vi "Periodic Tasks.vi"(8 "error in":errorcluster) -> ()   [LabVIEW 2018]
doc: "This VI runs in parallel to other tasks. It can contain as many user-defined periodic loops as you need. These can carry out PID or other sorts of timed response."
uses:
  CTL_RangeFinder_Type.ctl
  <vilib>/Rock Robotics/WPI/Utilities/WPI_GetSetVariantRefNum.vi
  Robot Global Data.vi
  <vilib>/Rock Robotics/Network Tables/NT Write Numeric Array.vi
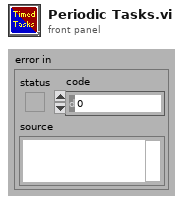
[diagram p1: front panel]
types:
  T1 = typedef "WPI_JoystickDevRef.ctl" = cluster{"Device":T2}
  T2 = typedef "WPI_JoystickDeviceEnum.ctl" = enum16{"USB 0", "USB 1", "USB 2", "USB 3", "USB 4", "USB 5"}
  T3 = typedef "WPI_RobotDriveDevRef.ctl" = cluster{"DevStatus":errorcluster, "Motors[]":T4[], "Square Inputs":bool, "Max Output":dbl}
  T4 = typedef "WPI_MotorControlDeviceRef.ctl" = cluster{"DeviceStatus":errorcluster, "Type":T5, "PWM":cluster{"PWM Channel":T6, "DeadBand":T7}, "CAN":cluster{"Device Number":u8, "SetOutput VI Ref":variant, "GetOutput VI Ref":variant, "Enable VI Ref":variant, "Disable VI Ref":variant, "Data":variant}, "Invert":bool, "DIO PWM":cluster{"PWM \"Enable\" Channel":T6, "DIOChannel":T8, "PWM Rate":dbl}}
  T5 = typedef "WPI_MotorControlType.ctl" = enum16{"PWM", "CAN", "DIO PWM"}
  T6 = typedef "FPGA_DIOPWMChannel.ctl" = enum8{"PWM 0", "PWM 1", "PWM 2", "PWM 3", "PWM 4", "PWM 5", "PWM 6", "PWM 7", "PWM 8", "PWM 9", "PWM MXP 0", "PWM MXP 1", "PWM MXP 2", "PWM MXP 3", "PWM MXP 4", "PWM MXP 5", "PWM MXP 6", "PWM MXP 7", "PWM MXP 8", "PWM MXP 9", "Invalid"}
  T7 = typedef "WPI_PWMDeadband.ctl" = cluster{"Name":string, "maxPositivePwm":i32, "minPositivePwm":i32, "centerPwm":i32, "maxNegativePwm":i32, "minNegativePwm":i32, "angularRange":u16}
  T8 = typedef "FPGA_DIOChannel.ctl" = enum8{"DIO 0", "DIO 1", "DIO 2", "DIO 3", "DIO 4", "DIO 5", "DIO 6", "DIO 7", "DIO 8", "DIO 9", "DIO MXP 0", "DIO MXP 1", "DIO MXP 2", "DIO MXP 3", "DIO MXP 4", "DIO MXP 5", "DIO MXP 6", "DIO MXP 7", "DIO MXP 8", "DIO MXP 9", "DIO MXP 10", "DIO MXP 11", "DIO MXP 12", "DIO MXP 13", "DIO MXP 14", "DIO MXP 15", "SPI Port CS1", "SPI Port CS2", "SPI Port CS3", "SPI Port MISO", "SPI Port MOSI", "Invalid"}
  T9 = cluster{"JoystickDevRef":T1, "RobotDriveDevRef":T3}
  T10 = typedef "CTL_RangeFinder_Type.ctl" = enum16{"GP2Y0A41SK0F (4-30)", "GP2Y0A02YK0F (20-150)", "GP2Y0A21YK0F (10-80)"}
  T11 = typedef "WPI_AnalogChannelDevRef.ctl" = cluster{"DevStatus":errorcluster, "Analog Channel":T12}
  T12 = typedef "FPGA_AIChannel.ctl" = enum8{"AI 0", "AI 1", "AI 2", "AI 3", "AI MXP 0", "AI MXP 1", "AI MXP 2", "AI MXP 3", "Invalid"}
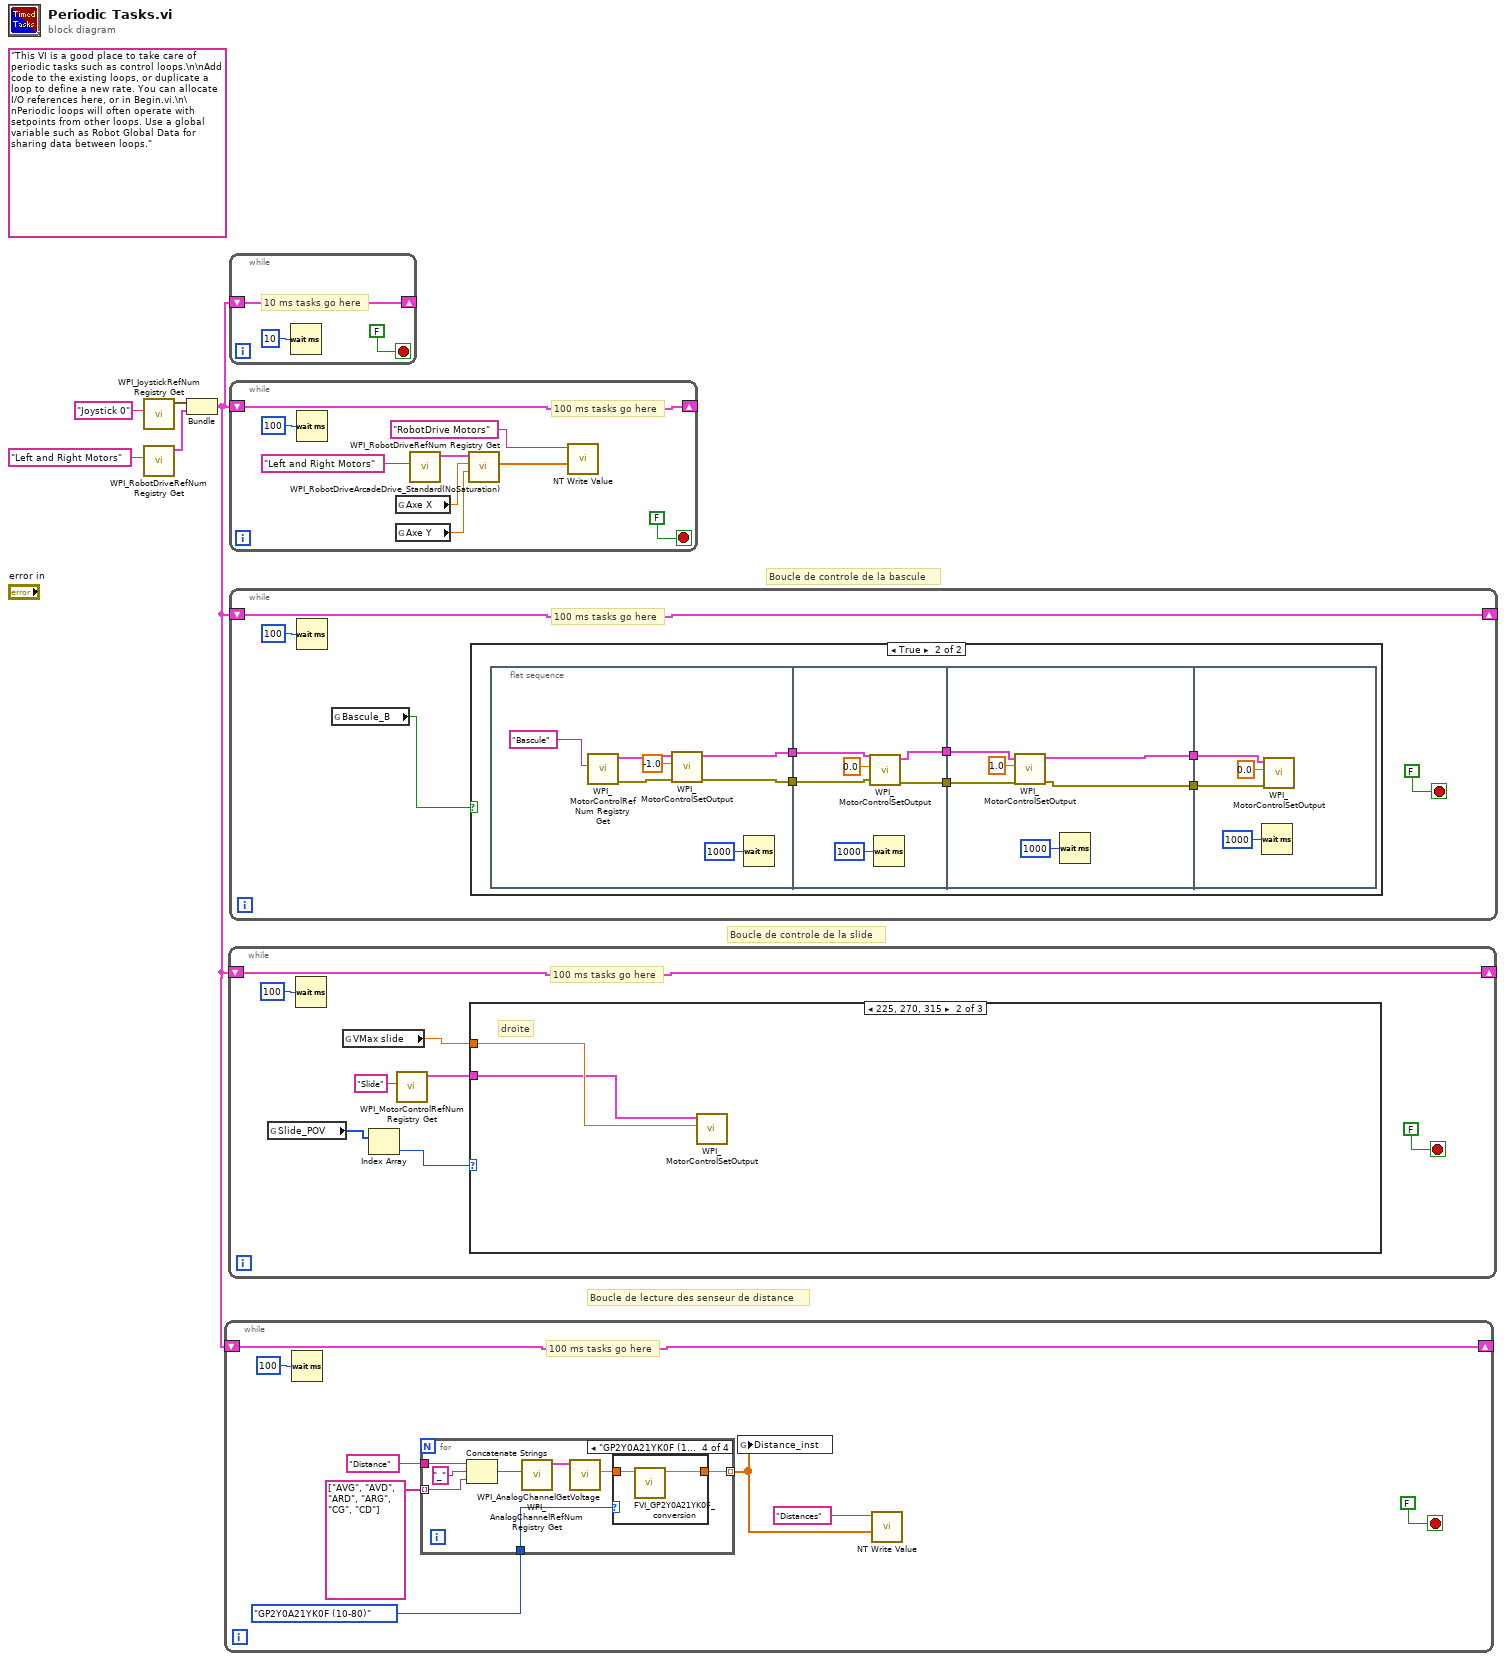
[diagram p0: block diagram]
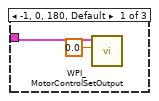
[diagram p5: hidden frame]
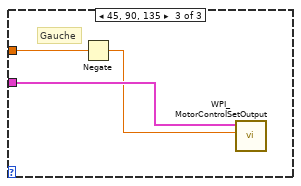
[diagram p6: hidden frame]
diagram:
  (unwired) "This VI is a good place to take care of periodic tasks such as control loops.\n\nAdd code to the existing loops, or duplicate a loop to define a new rate. You can allocate I/O references here, or in Begin.vi.\n\nPeriodic loops will often operate with setpoints from other loops. Use a global variable such as Robot Global Data for sharing data between loops."
  # "Boucle de lecture des senseur de distance"
  # "Boucle de controle de la slide"
  # "Boucle de controle de la bascule"
  n1 = call <vilib>:"WPI_JoystickRefNum Registry Get.vi"("refnum name"="Joystick 0") -> ("JoystickDevRef"=w3:T1)  [unwired: 1 in, 9 out]
  n2 = call <vilib>:"WPI_RobotDriveRefNum Registry Get.vi"("refnum name"="Left and Right Motors") -> ("RobotDriveDevRef"=w2:T3)  [unwired: 1 in, 9 out]
  n3 = Bundle("JoystickDevRef"=w3, "RobotDriveDevRef"=w2) -> (w1:T9)  [unwired: 1 out]
  n4 = while {
    shift-right: [w11] -> _
    shift-left: w1 -> [w11]
    stop <- FALSE stop-if-true
    # "100 ms tasks go here"
    n5 = Wait (ms)(milliseconds to wait=u32 100) -> ()  [unwired: 1 out]
    n6 = for {
      tunnel: "Distance" -> [w21]
      tunnel: string[] ["AVG", "AVD", "ARD", "ARG", "CG", "CD"] -> [w19] mode=indexing
      tunnel: [w15] -> w6 mode=indexing
      tunnel: CTL_RangeFinder_Type."GP2Y0A21YK0F (10-80)" ("Enum") -> [w14]
      n7 = Concatenate Strings(w21, "_" ("string"), w19) -> (w17:string)
      n8 = call <vilib>:"WPI_AnalogChannelRefNum Registry Get.vi"("refnum name"=w17) -> ("AIDeviceRef"=w18:T11)  [unwired: 9 in, 1 out]
      n9 = call <vilib>:"WPI_AnalogChannelGetVoltage.vi"("AIDeviceRef"=w18) -> ("Voltage"=w16:dbl)  [unwired: 8 in, 2 out]
      n10 = case shown="\"GP2Y0A21YK0F (10-80)\"" w14 {
        tunnel: w16 -> [w22 w23 w24 w26]
        tunnel: [w22 w23 w24 w25] -> w15
        frame "GP2Y0A41SK0F (4-30)" {
        }
        frame "GP2Y0A02YK0F (20-150)" {
        }
        frame Default {
        }
        frame "GP2Y0A21YK0F (10-80)" {
          n11 = call "FVI_GP2Y0A21YK0F_conversion.vi"("Voltage"=w26) -> ("Numeric"=w25:dbl)  [unwired: 10 in]
        }
      }
    }
    n12 = global write "Robot Global Data.vi" "Distance_inst"(w6) -> ()
    n13 = call-poly <vilib>:"NT Write Value.vi"("Numeric Array"=w6, "Name"="Distances") -> ()  [unwired: 9 in, 1 out]
  }
  n14 = while {
    shift-right: [w32] -> _
    shift-left: w1 -> [w32]
    stop <- FALSE stop-if-true
    # "100 ms tasks go here"
    n15 = global read "Robot Global Data.vi" "Slide_POV"() -> (w31:i16[])
    n16 = Wait (ms)(milliseconds to wait=u32 100) -> ()  [unwired: 1 out]
    n17 = global read "Robot Global Data.vi" "VMax slide"() -> (w27:dbl)
    n18 = Index Array(array=w31) -> (element=w30:i16)  [unwired: 1 in]
    n19 = call <vilib>:"WPI_MotorControlRefNum Registry Get.vi"("refnum name"="Slide") -> ("MotorControlDevRef"=w28:T4)  [unwired: 9 in, 1 out]
    n20 = case shown="225, 270, 315" w30 {
      tunnel: w28 -> [w36 w37 w40]
      tunnel: w27 -> [_ w38 w41]
      frame -1, 0, 180, Default {
        n21 = call <vilib>:"WPI_MotorControlSetOutput.vi"("Output"=0.0, "MotorControlDevRef"=w36) -> ()  [unwired: 7 in, 3 out]
      }
      frame 225, 270, 315 {
        # "droite"
        n22 = call <vilib>:"WPI_MotorControlSetOutput.vi"("Output"=w38, "MotorControlDevRef"=w37) -> ()  [unwired: 7 in, 3 out]
      }
      frame 45, 90, 135 {
        # "Gauche"
        n23 = Negate(x=w41) -> (-x=w39:dbl)
        n24 = call <vilib>:"WPI_MotorControlSetOutput.vi"("Output"=w39, "MotorControlDevRef"=w40) -> ()  [unwired: 7 in, 3 out]
      }
    }
  }
  n25 = while {
    shift-right: [w42] -> _
    shift-left: w1 -> [w42]
    stop <- FALSE stop-if-true
    # "10 ms tasks go here"
    n26 = Wait (ms)(milliseconds to wait=u32 10) -> ()  [unwired: 1 out]
  }
  n27 = while {
    shift-right: [w51] -> _
    shift-left: w1 -> [w51]
    stop <- FALSE stop-if-true
    # "100 ms tasks go here"
    n28 = Wait (ms)(milliseconds to wait=u32 100) -> ()  [unwired: 1 out]
    n29 = global read "Robot Global Data.vi" "Axe X"() -> (w45:dbl)
    n30 = global read "Robot Global Data.vi" "Axe Y"() -> (w46:dbl)
    n31 = call <vilib>:"WPI_RobotDriveRefNum Registry Get.vi"("refnum name"="Left and Right Motors") -> ("RobotDriveDevRef"=w49:T3)  [unwired: 1 in, 9 out]
    n32 = call <vilib>:"WPI_RobotDriveArcadeDrive_Standard(NoSaturation).vi"("Y axis value"=w46, "X axis value"=w45, "RobotDriveDevRef"=w49) -> ("Motor Values"=w48:dbl[])  [unwired: 1 in, 7 out]
    n33 = call-poly <vilib>:"NT Write Value.vi"("Numeric Array"=w48, "Name"="RobotDrive Motors") -> ()  [unwired: 9 in, 1 out]
  }
  n34 = while {
    shift-right: [w55] -> _
    shift-left: w1 -> [w55]
    stop <- FALSE stop-if-true
    # "100 ms tasks go here"
    n35 = Wait (ms)(milliseconds to wait=u32 100) -> ()  [unwired: 1 out]
    n36 = global read "Robot Global Data.vi" "Bascule_B"() -> (w54:bool)
    n37 = case shown="True" w54 {
      frame False {
      }
      frame True {
        n38 = flat-sequence {
          tunnel: [w66] -> w63
          tunnel: [w65] -> w60
          tunnel: w63 -> [w75]
          tunnel: [w74] -> w62
          tunnel: w60 -> [w73]
          tunnel: [w72] -> w59
          tunnel: w62 -> [w81]
          tunnel: [w80] -> w61
          tunnel: w59 -> [w79]
          tunnel: [w78] -> w58
          tunnel: w61 -> [w85]
          tunnel: w58 -> [w84]
          frame #0 {
            n39 = call <vilib>:"WPI_MotorControlRefNum Registry Get.vi"("refnum name"="Bascule") -> ("error out"=w69:errorcluster, "MotorControlDevRef"=w70:T4)  [unwired: 9 in]
            n40 = call <vilib>:"WPI_MotorControlSetOutput.vi"("error in (no error)"=w69, "Output"=-1.0, "MotorControlDevRef"=w70) -> ("error out"=w65:errorcluster, "MotorControlDevRef"=w66:T4)  [unwired: 6 in, 1 out]
            n41 = Wait (ms)(milliseconds to wait=u32 1000) -> ()  [unwired: 1 out]
          }
          frame #1 {
            n42 = call <vilib>:"WPI_MotorControlSetOutput.vi"("error in (no error)"=w73, "Output"=0.0, "MotorControlDevRef"=w75) -> ("error out"=w72:errorcluster, "MotorControlDevRef"=w74:T4)  [unwired: 6 in, 1 out]
            n43 = Wait (ms)(milliseconds to wait=u32 1000) -> ()  [unwired: 1 out]
          }
          frame #2 {
            n44 = call <vilib>:"WPI_MotorControlSetOutput.vi"("error in (no error)"=w79, "Output"=1.0, "MotorControlDevRef"=w81) -> ("error out"=w78:errorcluster, "MotorControlDevRef"=w80:T4)  [unwired: 6 in, 1 out]
            n45 = Wait (ms)(milliseconds to wait=u32 1000) -> ()  [unwired: 1 out]
          }
          frame #3 {
            n46 = Wait (ms)(milliseconds to wait=u32 1000) -> ()  [unwired: 1 out]
            n47 = call <vilib>:"WPI_MotorControlSetOutput.vi"("error in (no error)"=w84, "Output"=0.0, "MotorControlDevRef"=w85) -> ()  [unwired: 6 in, 3 out]
          }
        }
      }
    }
  }
